vi "TopLevel_Ref_FGV.vi"(6 "Action":enum16{"Get", "Set", "Init"}(ring), 11 "TopLevel In":refnum<class "TopLevel.lvclass">) -> (3 "TopLevel Out":refnum<class "TopLevel.lvclass">)   [LabVIEW 2022 SP3, in "TopLevel.lvclass"]
uses:
  TopLevel.lvclass
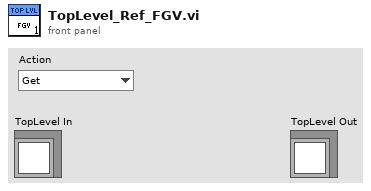
[diagram p1: front panel]
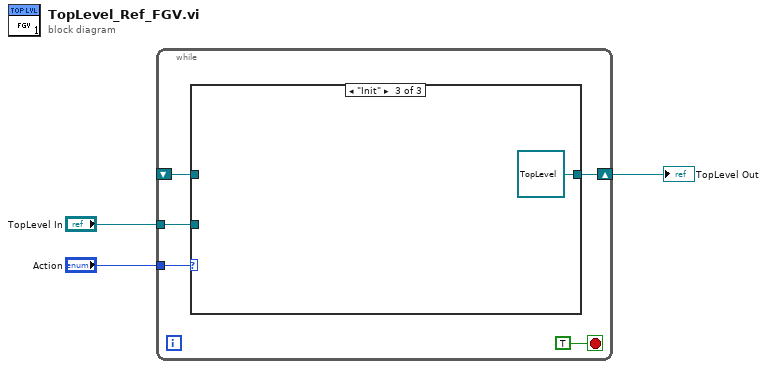
[diagram p0: block diagram]
diagram:
  n1 = while {
    tunnel: "Action" -> [w7]
    shift-right: [w5] -> w2
    shift-left: _ -> [w6]
    tunnel: "TopLevel In" -> [w4]
    stop <- TRUE stop-if-true
    n2 = case shown="\"Init\"" w7 {
      tunnel: w6 -> [w9 _ _]
      tunnel: [w9 w10 refnum<class "TopLevel.lvclass"> refnum ("TopLevel In")] -> w5
      tunnel: w4 -> [_ w10 _]
      frame "Get" {
      }
      frame "Set" {
      }
      frame "Init" {
      }
    }
  }
  "TopLevel Out" <- w2
